vi "No Internet Connection--error.vi"() -> (0 "error out":errorcluster)   [LabVIEW 2020, in "SimpleDependencyInspector.lvlib"]
uses:
  SimpleDependencyInspector.lvlib
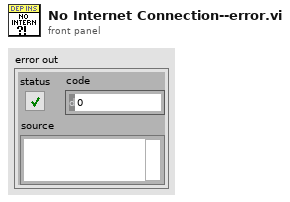
[diagram p1: front panel]
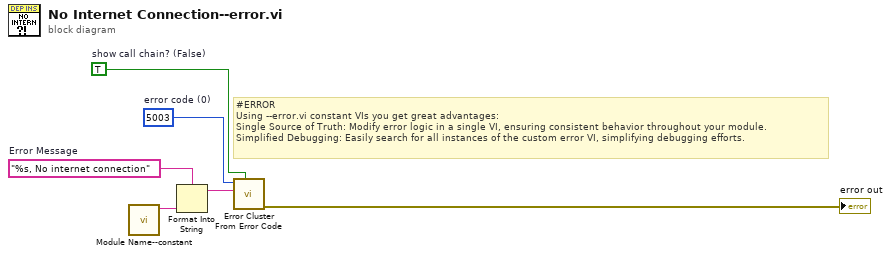
[diagram p0: block diagram]
diagram:
  w4 = 5003  # error code (0)
  w1 = "%s, No internet connection"  # Error Message
  w5 = TRUE  # show call chain? (False)
  # "#ERROR\nUsing --error.vi constant VIs you get great advantages:\nSingle Source of Truth: Modify error logic in a single VI, ensuring consistent behavior throughout your module.\nSimplified Debugging: Easily search for all instances of the custom error VI, simplifying debugging efforts."
  n1 = call "Module Name--constant.vi"() -> ("Module Name"=w3:string)  [unwired: 11 in]
  n2 = Format Into String(format string=w1, w3) -> (resulting string=w2:string)  [unwired: 2 in, 1 out]
  n3 = call <vilib>:"Error Cluster From Error Code.vi"("show call chain? (False)"=w5, "error message (\"\")"=w2, "error code (0)"=w4) -> ("error out"=→"error out":errorcluster)  [unwired: 6 in]
